vi "Get Simplified Image.vi"(8 "error in (no error)":errorcluster, 9 "Hide Grid?":bool, 11 "Sub VI Ref":refnum<vi>) -> (0 "error out":errorcluster, 1 "bounds":T1, 2 "new picture":picture, 3 "Dup Sub VI Ref":refnum<vi>)   [LabVIEW 2017, in "XY Plot Matrix.lvclass"]
uses:
  <vilib>/Math Plots/2D Math Plots/XY Plot Matrix/XY Plot Matrix/XY Plot Matrix.lvclass
  <vilib>/picture/picture.llb/imagedata.ctl
  <vilib>/Utility/miscctls.llb/LVBoundsTypeDef.ctl
  <vilib>/Math Plots/Plot Private Lib/NI_Math Plot Private Lib.lvlib
panel:
  in  "image data":T2
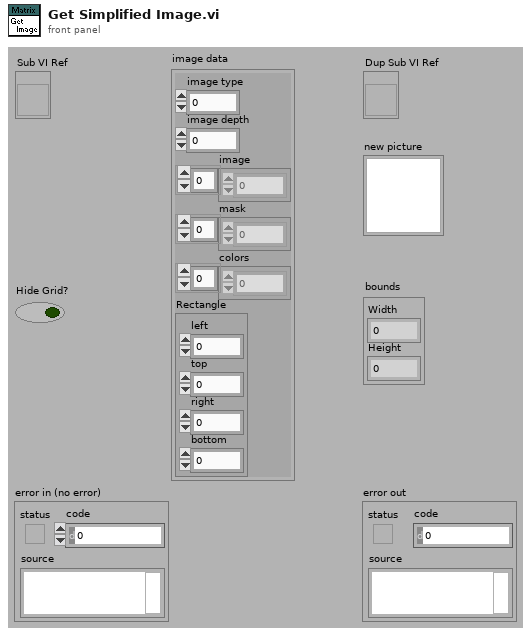
[diagram p1: front panel]
types:
  T1 = typedef "LVBoundsTypeDef.ctl" = cluster{"Width":u32, "Height":u32}
  T2 = typedef "imagedata.ctl" = cluster{"image type":i32, "image depth":i32, "image":u8[], "mask":u8[], "colors":u32[], "Rectangle":cluster{"left":i16, "top":i16, "right":i16, "bottom":i16}}
  T3 = typedef "LVRectTypeDef.ctl" = cluster{"Left":i16, "Top":i16, "Right":i16, "Bottom":i16}
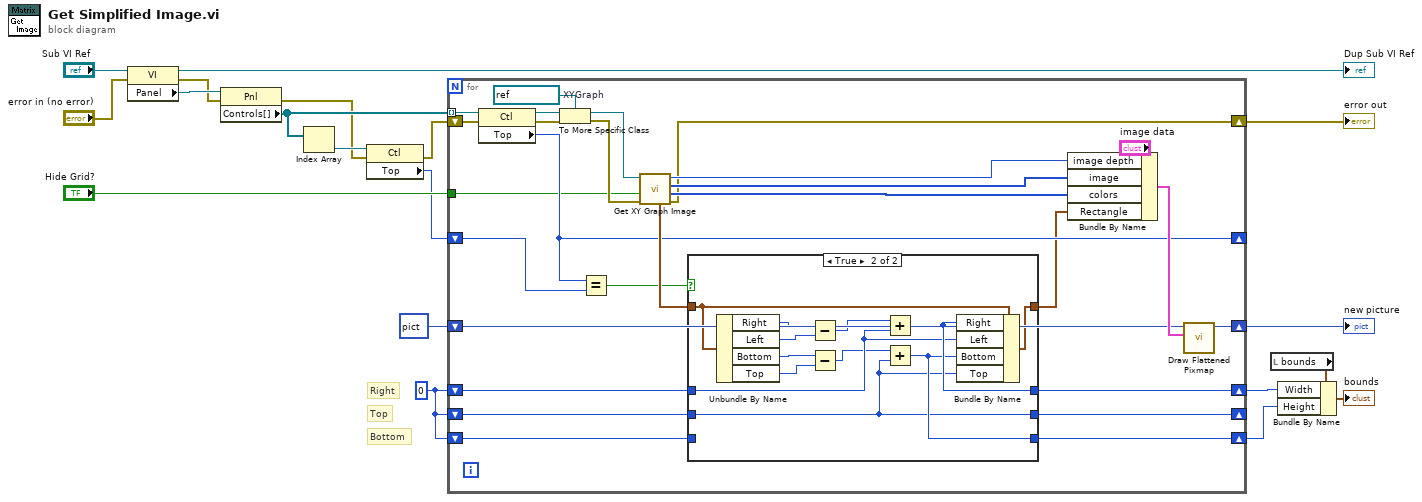
[diagram p0: block diagram]
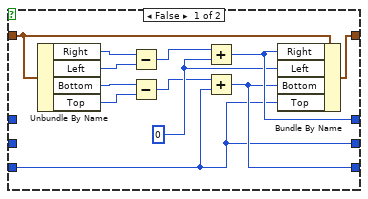
[diagram p2: hidden frame]
diagram:
  w5 = i16 0 ("Position:Top")
  # "Top"
  # "Bottom"
  # "Right"
  n1 = property class="VI"(reference="Sub VI Ref", error in="error in (no error)") -> (reference out=→"Dup Sub VI Ref":refnum<vi>, error out=w15:errorcluster, "Panel"=w18:refnum<vi>)
  n2 = property class="Pnl"(reference=w18, error in=w15) -> (error out=w8:errorcluster, "Controls[]"=w10:refnum<vi>[])  [unwired: 1 out]
  n3 = Index Array(array=w10) -> (element=w9:refnum<vi>)  [unwired: 1 in]
  n4 = property class="Ctl"(reference=w9, error in=w8) -> (error out=w7:errorcluster, "Top"=w6:i32)  [unwired: 1 out]
  n5 = for {
    tunnel: w10 -> [w40] mode=indexing
    tunnel: "Hide Grid?" -> [w20]
    shift-right: [w36] -> w12
    shift-left: w7 -> [w41]
    shift-right: [w35] -> w13
    shift-left: picture data[5B] ("new picture") -> [w34]
    shift-right: [w31] -> _
    shift-left: w6 -> [w32]
    shift-right: [w26] -> w3
    shift-left: w5 -> [w29]
    shift-right: [w25] -> w2
    shift-left: w5 -> [w28]
    shift-right: [w24] -> _
    shift-left: w5 -> [w23]
    w39 = refnum<vi> refnum  # XYGraph
    n6 = property class="Ctl"(reference=w40, error in=w41) -> (reference out=w38:refnum<vi>, error out=w37:errorcluster, "Top"=w31:i32)
    n7 = To More Specific Class(target class=w39, reference=w38, error in=w37) -> (specific class reference=w21:refnum<vi>, error out=w22:errorcluster)
    n8 = Equal?(x=w31, y=w32) -> (x = y?=w30:bool)
    n9 = call <vilib>:"Get XY Graph Image.vi"("error in (no error)"=w22, "Hide Grid?"=w20, "XY Graph Ref"=w21) -> ("error out"=w36:errorcluster, "Colors"=w45:u32[], "Image"=w44:u8[], "Image Depth"=w42:i32, "Bounds"=w33:T3)  [unwired: 4 out]
    n10 = case shown="True" w30 {
      tunnel: w33 -> [w55 w68]
      tunnel: w29 -> [_ w64]
      tunnel: w28 -> [w47 _]
      tunnel: [w54 w66] -> w27
      tunnel: [w53 w65] -> w26
      tunnel: [w48 w60] -> w25
      tunnel: [w47 w59] -> w24
      tunnel: w23 -> [_ w59]
      frame False {
        w52 = i16 0 ("Position:Top")
        n11 = Unbundle By Name(w55) -> ("Right"=w58:i16, "Left"=w57:i16, "Bottom"=w51:i16, "Top"=w50:i16)
        n12 = Subtract(x=w58, y=w57) -> (x-y=w56:i16)
        n13 = Subtract(x=w51, y=w50) -> (x-y=w49:i16)
        n14 = Add(x=w56, y=w52) -> (x+y=w53:i16)
        n15 = Add(x=w49, y=w47) -> (x+y=w48:i16)
        n16 = Bundle By Name(cluster=w55, "Right"=w53, "Left"=w52, "Bottom"=w48, "Top"=w47) -> (w54:T3)
      }
      frame True {
        n17 = Unbundle By Name(w68) -> ("Right"=w70:i16, "Left"=w69:i16, "Bottom"=w63:i16, "Top"=w62:i16)
        n18 = Subtract(x=w70, y=w69) -> (x-y=w67:i16)
        n19 = Subtract(x=w63, y=w62) -> (x-y=w61:i16)
        n20 = Add(x=w67, y=w64) -> (x+y=w65:i16)
        n21 = Add(x=w61, y=w59) -> (x+y=w60:i16)
        n22 = Bundle By Name(cluster=w68, "Right"=w65, "Left"=w64, "Bottom"=w60, "Top"=w59) -> (w66:T3)
      }
    }
    n23 = Bundle By Name(cluster="image data", "image depth"=w42, "image"=w44, "colors"=w45, "Rectangle"=w27) -> (w43:T2)
    n24 = call <vilib>:"Draw Flattened Pixmap.vi"("image data"=w43, "picture"=w34) -> ("new picture"=w35:picture)  [unwired: 7 out]
  }
  "error out" <- w12
  "new picture" <- w13
  n25 = local read "bounds"() -> (w4:T1)
  n26 = Bundle By Name(cluster=w4, "Width"=w3, "Height"=w2) -> (→"bounds":T1)
